vi "PWM Waveform Analysis - DG.vi"(0 "Analysis Leg":i32, 1 "Board Selector":T1, 5 "Active Leg":i32, 7 "Duty Cycle":i32=25, 9 "Waveform":waveform(dbl)[](array[waveform])) -> (4 "Active Leg Actual Duty":dbl, 10 "Result (Boolean)":bool, 15 "Message":string)   [LabVIEW 2022 SP3]
uses:
  Serial Board Com/Board Select.ctl
  <vilib>/measure/mascope.llb/Pulse Measurements 1 chan.vi
  <vilib>/measure/madcrms.llb/Basic Averaged DC-RMS for 1 Chan.vi
  <vilib>/measure/NI_MAPro.lvlib
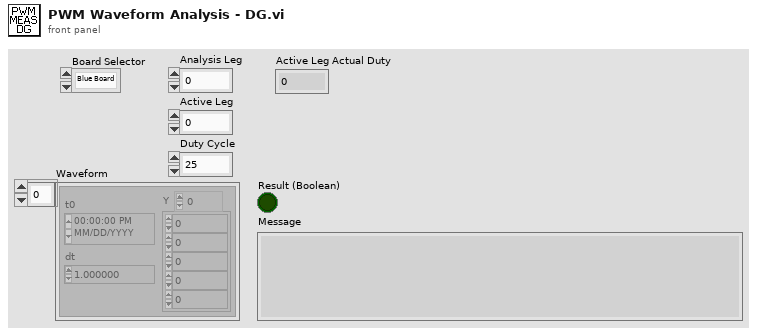
[diagram p1: front panel]
types:
  T1 = typedef "Board Select.ctl" = enum16{"Blue Board", "Green Board"}
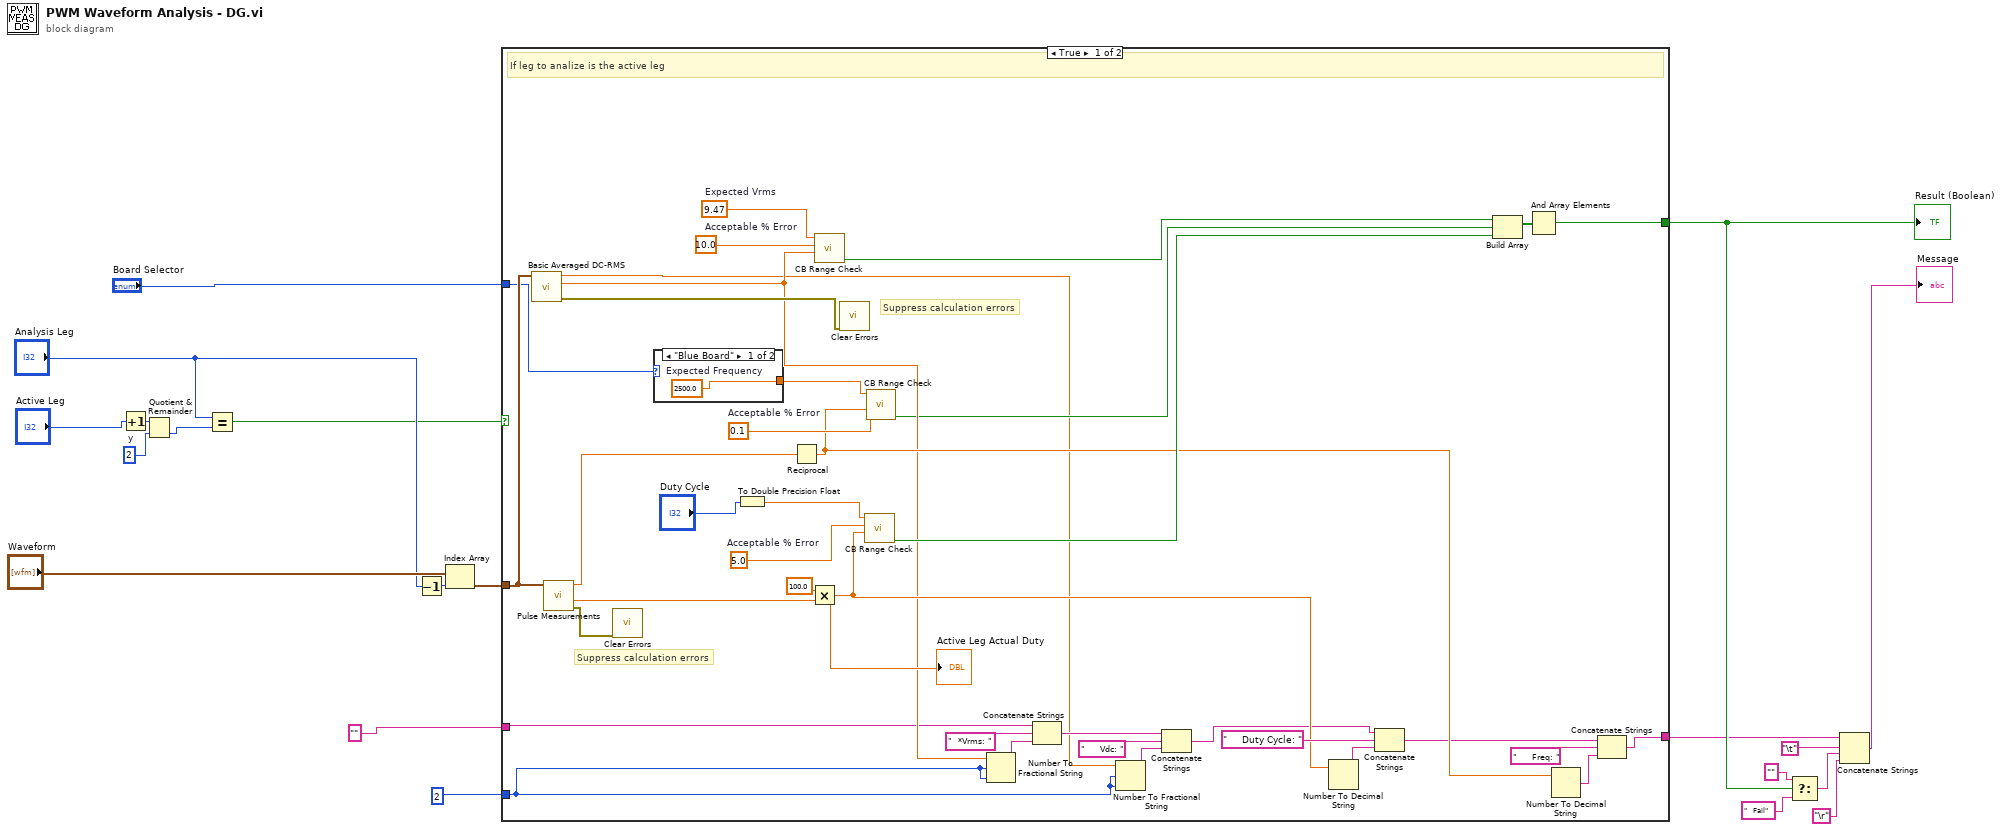
[diagram p0: block diagram]
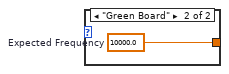
[diagram p2: hidden frame]
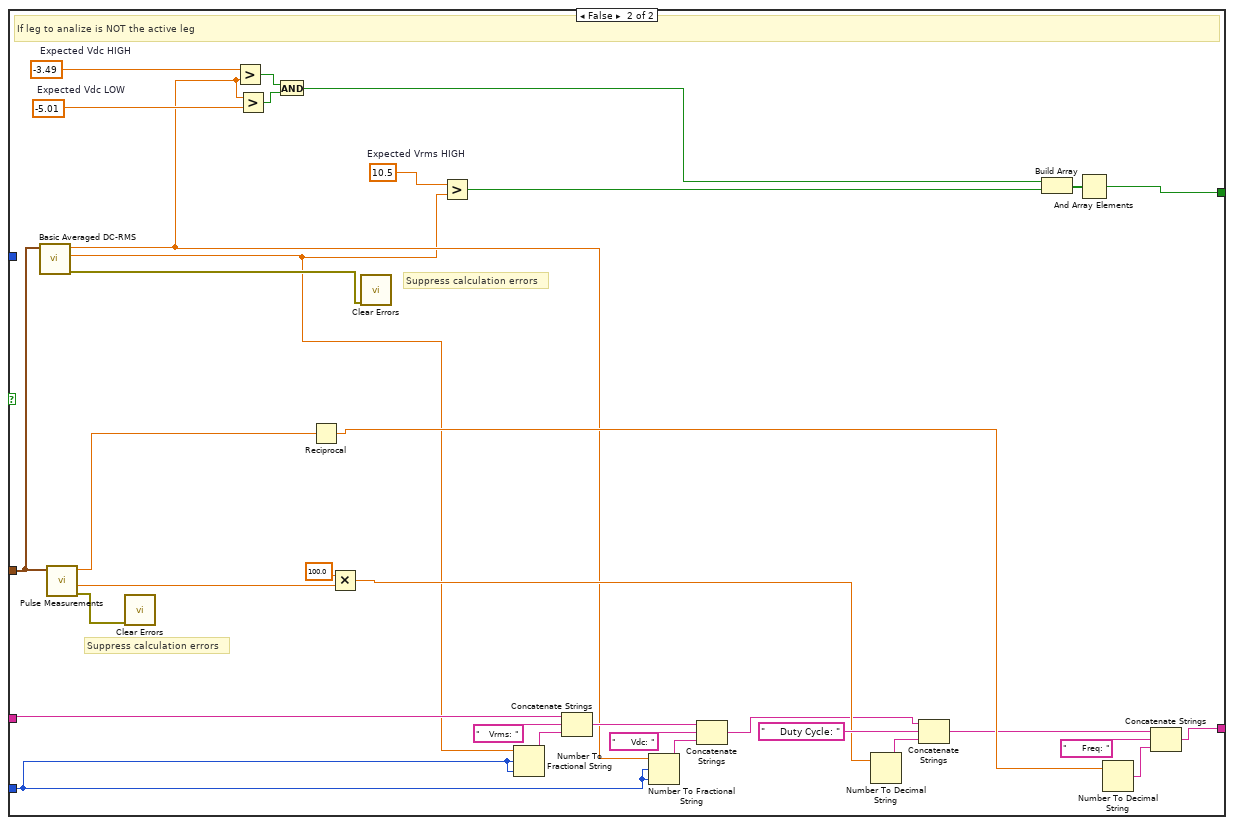
[diagram p3: hidden frame]
diagram:
  w5 = 2  # y
  n1 = Increment(x="Active Leg") -> (x+1=w4:i32)
  n2 = Quotient & Remainder(x=w4, y=w5) -> (floor(x/y)=w3:i32)  [unwired: 1 out]
  n3 = Equal?(x="Analysis Leg", y=w3) -> (x = y?=w9:bool)
  n4 = Decrement(x="Analysis Leg") -> (x-1=w20:i32)
  n5 = Index Array(array="Waveform", index=w20) -> (element=w15:waveform(dbl))
  n6 = case shown="True" w9 {
    tunnel: w15 -> [w42 w80]
    tunnel: [w36 w77] -> w11
    tunnel: [w26 w65] -> w10
    tunnel: "" -> [w28 w67]
    tunnel: 2 -> [w25 w64]
    tunnel: "Board Selector" -> [w21 _]
    frame True {
      w31 = 10.0  # Acceptable % Error
      w30 = 9.47  # Expected Vrms
      w50 = 5.0  # Acceptable % Error
      w51 = 0.1  # Acceptable % Error
      # "Suppress calculation errors"
      # "Suppress calculation errors"
      # "If leg to analize is the active leg"
      n7 = call-poly <vilib>:"Basic Averaged DC-RMS.vi"("signal in"=w42) -> ("error out"=w43:errorcluster, "RMS value"=w38:dbl, "DC value"=w29:dbl)  [unwired: 7 in, 1 out]
      n8 = call-poly <vilib>:"Pulse Measurements.vi"("signal in"=w42) -> ("error out"=w52:errorcluster, "duty cycle"=w54:dbl, "period"=w53:dbl)  [unwired: 6 in, 2 out]
      n9 = call <vilib>:"Clear Errors.vi"("error in (no error)"=w52) -> ()  [unwired: 5 in, 2 out]
      n10 = case shown="\"Blue Board\"" w21 {
        tunnel: [w58 w59] -> w22
        frame "Blue Board" {
          w58 = 2500.0  # Expected Frequency
        }
        frame "Green Board" {
          w59 = 10000.0  # Expected Frequency
        }
      }
      n11 = To Double Precision Float(number="Duty Cycle") -> (double precision float=w23:dbl)
      n12 = Reciprocal(x=w53) -> (1/x=w44:dbl)
      n13 = Multiply(x=100.0, y=w54) -> (x*y=w47:dbl)
      "Active Leg Actual Duty" <- w47
      n14 = call "CB Range Check.vi"("Actual Value"=w38, "Acceptable% Error"=w31, "Expected Value"=w30) -> ("Result (Boolean)"=w41:bool)  [unwired: 6 in, 2 out]
      n15 = call <vilib>:"Clear Errors.vi"("error in (no error)"=w43) -> ()  [unwired: 5 in, 2 out]
      n16 = call "CB Range Check.vi"("Actual Value"=w47, "Acceptable% Error"=w50, "Expected Value"=w23) -> ("Result (Boolean)"=w55:bool)  [unwired: 6 in, 2 out]
      n17 = call "CB Range Check.vi"("Actual Value"=w44, "Acceptable% Error"=w51, "Expected Value"=w22) -> ("Result (Boolean)"=w37:bool)  [unwired: 6 in, 2 out]
      n18 = Number To Fractional String(number=w38, width (-)=w25, precision (6)=w25) -> (F-format string=w40:string)  [unwired: 1 in]
      n19 = Concatenate Strings(w28, "  *Vrms: " ("string"), w40) -> (w32:string)
      n20 = Number To Fractional String(number=w29, width (-)=w25, precision (6)=w25) -> (F-format string=w34:string)  [unwired: 1 in]
      n21 = Concatenate Strings(w32, "     Vdc: " ("string"), w34) -> (w27:string)
      n22 = Number To Decimal String(number=w47) -> (decimal integer string=w48:string)  [unwired: 1 in]
      n23 = Concatenate Strings(w27, "     Duty Cycle: " ("string"), w48) -> (w33:string)
      n24 = Build Array(w41, w37, w55) -> (w56:bool[])
      n25 = And Array Elements(Boolean array=w56) -> (logical AND=w36:bool)
      n26 = Number To Decimal String(number=w44) -> (decimal integer string=w45:string)  [unwired: 1 in]
      n27 = Concatenate Strings(w33, "     Freq: " ("string"), w45) -> (w26:string)
    }
    frame False {
      w63 = 10.5  # Expected Vrms HIGH
      w71 = -5.01  # Expected Vdc LOW
      w72 = -3.49  # Expected Vdc HIGH
      # "Suppress calculation errors"
      # "Suppress calculation errors"
      # "If leg to analize is NOT the active leg"
      n28 = call-poly <vilib>:"Basic Averaged DC-RMS.vi"("signal in"=w80) -> ("error out"=w81:errorcluster, "RMS value"=w62:dbl, "DC value"=w68:dbl)  [unwired: 7 in, 1 out]
      n29 = call-poly <vilib>:"Pulse Measurements.vi"("signal in"=w80) -> ("error out"=w88:errorcluster, "duty cycle"=w90:dbl, "period"=w89:dbl)  [unwired: 6 in, 2 out]
      n30 = call <vilib>:"Clear Errors.vi"("error in (no error)"=w88) -> ()  [unwired: 5 in, 2 out]
      n31 = Greater?(x=w72, y=w68) -> (0:w70:bool)
      n32 = Greater?(x=w68, y=w71) -> (0:w69:bool)
      n33 = And(x=w70, y=w69) -> (x .and. y?=w60:bool)
      n34 = Reciprocal(x=w89) -> (1/x=w82:dbl)
      n35 = Multiply(x=100.0, y=w90) -> (x*y=w85:dbl)
      n36 = call <vilib>:"Clear Errors.vi"("error in (no error)"=w81) -> ()  [unwired: 5 in, 2 out]
      n37 = Greater?(x=w63, y=w62) -> (0:w61:bool)
      n38 = Number To Fractional String(number=w62, width (-)=w64, precision (6)=w64) -> (F-format string=w79:string)  [unwired: 1 in]
      n39 = Concatenate Strings(w67, "   Vrms: " ("string"), w79) -> (w73:string)
      n40 = Number To Fractional String(number=w68, width (-)=w64, precision (6)=w64) -> (F-format string=w75:string)  [unwired: 1 in]
      n41 = Concatenate Strings(w73, "     Vdc: " ("string"), w75) -> (w66:string)
      n42 = Number To Decimal String(number=w85) -> (decimal integer string=w86:string)  [unwired: 1 in]
      n43 = Concatenate Strings(w66, "     Duty Cycle: " ("string"), w86) -> (w74:string)
      n44 = Build Array(w60, w61) -> (w91:bool[])
      n45 = And Array Elements(Boolean array=w91) -> (logical AND=w77:bool)
      n46 = Number To Decimal String(number=w82) -> (decimal integer string=w83:string)  [unwired: 1 in]
      n47 = Concatenate Strings(w74, "     Freq: " ("string"), w83) -> (w65:string)
    }
  }
  "Result (Boolean)" <- w11
  n48 = Select(t="" ("string"), s=w11, f="   Fail" ("string")) -> (s? t:f=w12:string)
  n49 = Concatenate Strings(w10, "\t", w12, "\r") -> (→"Message":string)
